vi "get_pressure_gauge_readings (SubVI).vi"(8 "error in":errorcluster, 11 "pressure_gauge_monitors":tag="Dev3/ai3,Dev3/ai6,Dev3/ai14") -> (0 "error out":errorcluster, 1 "baratron":dbl=0.021272970096496462 format="%0.2f", 2 "1torr_baratron":dbl=0.10636485048248231 format="%0.2f", 3 "pirani":dbl=7.448668533104113 format="%0.2f")   [LabVIEW 2022 SP3]
uses:
  <vilib>/DAQmx/read.llb/DAQmx Read (Analog 2D DBL NChan NSamp).vi
  <vilib>/Analysis/baseanly.llb/Mean (DBL).vi
  <vilib>/DAQmx/create/channels.llb/DAQmx Create Channel (AI-Voltage-Basic).vi
  <vilib>/DAQmx/configure/timing.llb/DAQmx Timing (Sample Clock).vi
  <vilib>/DAQmx/miscellaneous.llb/DAQmx Fill In Error Info.vi
  <vilib>/Analysis/NI_AALBase.lvlib
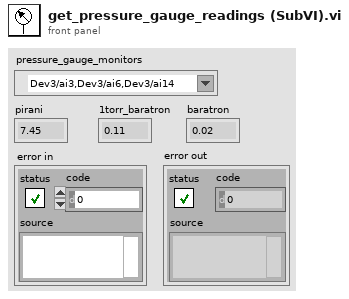
[diagram p1: front panel]
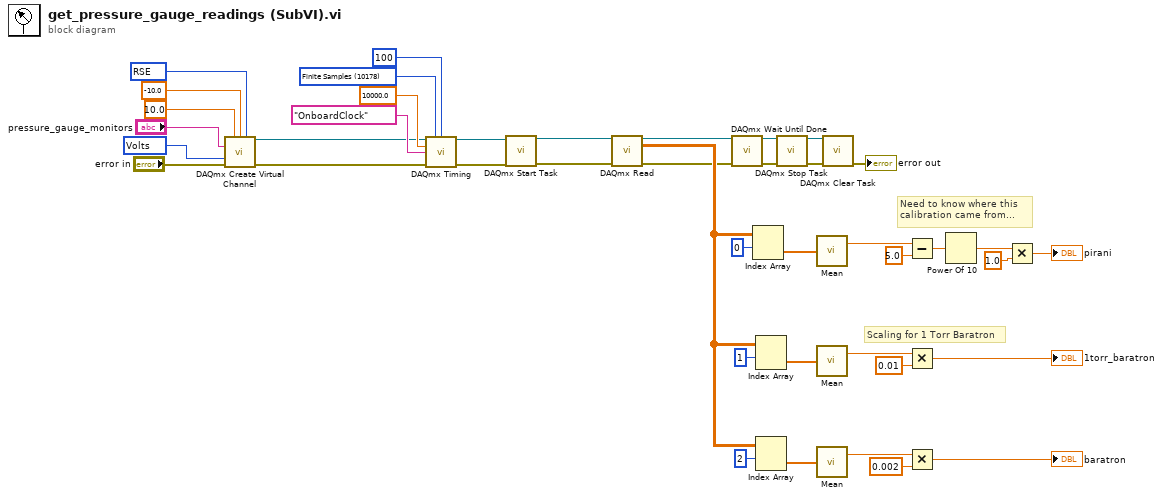
[diagram p0: block diagram]
diagram:
  w25 = 10178 items=["Finite Samples"=10178, "Continuous Samples"=10123, "Hardware Timed Single Point"=12522] ("sample mode")
  w37 = 10083 items=["default"=-1, "RSE"=10083, "NRSE"=10078, "Differential"=10106, "Pseudodifferential"=12529] ("input terminal configuration")
  w39 = 10348 items=["Volts"=10348, "From Custom Scale"=10065] ("units")
  # "Scaling for 1 Torr Baratron"
  # "Need to know where this\ncalibration came from..."
  n1 = call-poly <vilib>:"DAQmx Create Virtual Channel.vi"("maximum value"=10.0, "minimum value"=-10.0, "input terminal configuration"=w37, "physical channels"="pressure_gauge_monitors", "units"=w39, "error in"="error in") -> ("task out"=w23:refnum<k21>, "error out"=w22:errorcluster)  [unwired: 8 in]
  n2 = call-poly <vilib>:"DAQmx Timing.vi"("task/channels in"=w23, "sample mode"=w25, "samples per channel"=100, "rate"=10000.0, "source"=tag "OnboardClock", "error in"=w22) -> ("task out"=w21:refnum<k21>, "error out"=w20:errorcluster)  [unwired: 8 in]
  n3 = call <vilib>:"DAQmx Start Task.vi"("task/channels in"=w21, "error in"=w20) -> ("task out"=w38:refnum<k21>, "error out"=w32:errorcluster)  [unwired: 12 in]
  n4 = call-poly <vilib>:"DAQmx Read.vi"("task/channels in"=w38, "error in"=w32) -> ("task out"=w18:refnum<k21>, "data"=w33:dbl[][], "error out"=w17:errorcluster)  [unwired: 11 in]
  n5 = call <vilib>:"DAQmx Wait Until Done.vi"("task/channels in"=w18, "error in"=w17) -> ("task out"=w16:refnum<k21>, "error out"=w15:errorcluster)  [unwired: 12 in]
  n6 = Index Array(array=w33, index (row)=0 ("index")) -> (element=w30:dbl[])  [unwired: 1 in]
  n7 = Index Array(array=w33, index (row)=1 ("index")) -> (element=w29:dbl[])  [unwired: 1 in]
  n8 = Index Array(array=w33, index (row)=2 ("index")) -> (element=w28:dbl[])  [unwired: 1 in]
  n9 = call <vilib>:"DAQmx Stop Task.vi"("task/channels in"=w16, "error in"=w15) -> ("task out"=w14:refnum<k21>, "error out"=w13:errorcluster)  [unwired: 12 in]
  n10 = call-poly <vilib>:"Mean.vi"("X"=w30) -> ("mean"=w8:dbl)  [unwired: 1 out]
  n11 = call-poly <vilib>:"Mean.vi"("X"=w29) -> ("mean"=w5:dbl)  [unwired: 1 out]
  n12 = call-poly <vilib>:"Mean.vi"("X"=w28) -> ("mean"=w2:dbl)  [unwired: 1 out]
  n13 = call <vilib>:"DAQmx Clear Task.vi"("task in"=w14, "error in"=w13) -> ("error out"=→"error out":errorcluster)  [unwired: 13 in]
  n14 = Subtract(x=w8, y=5.0) -> (x-y=w11:dbl)
  n15 = Multiply(x=w5, y=0.01) -> (x*y=→"1torr_baratron":dbl)
  n16 = Multiply(x=w2, y=0.002) -> (x*y=→"baratron":dbl)
  n17 = Power Of 10(x=w11) -> (10^x=w10:dbl)
  n18 = Multiply(x=w10, y=1.0) -> (x*y=→"pirani":dbl)
